vi "_interfacebrowser Build Interface Menu.vi"(5 "Tree":refnum<vi>, 7 "CtlRef":refnum<vi>, 9 "Coords":T1, 11 "Menu in":refnum<k9>) -> (3 "Discard?":bool)   [LabVIEW 2017, in "interfacebrowser.lvlib"]
uses:
  interfacebrowser.lvlib
  <vilib>/Utility/miscctls.llb/LVPoint32TypeDef.ctl
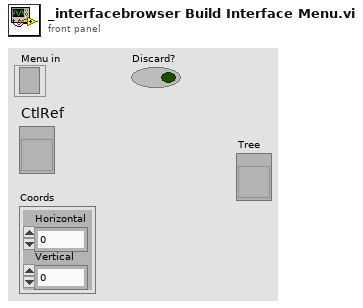
[diagram p1: front panel]
types:
  T1 = typedef "LVPoint32TypeDef.ctl" = cluster{"Horizontal":i32, "Vertical":i32}
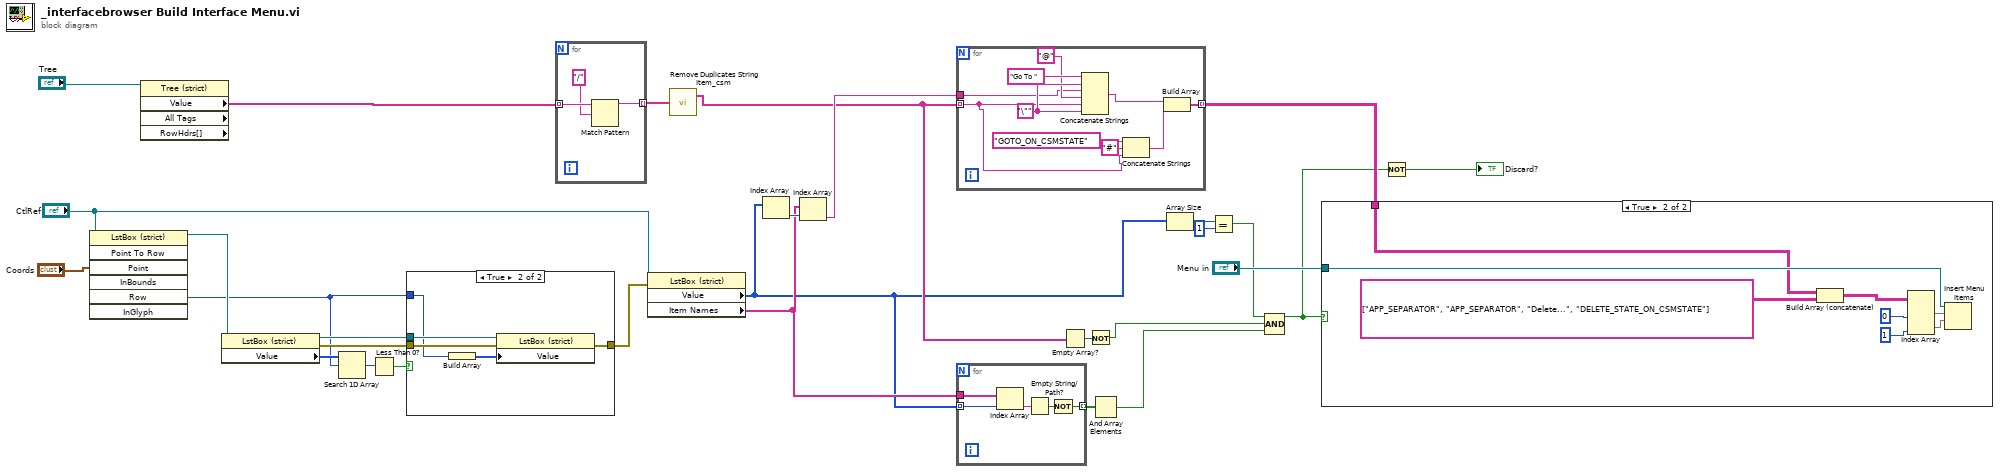
[diagram p0: block diagram]
diagram:
  n1 = invoke on="Invoke Node" class="LstBox (strict)" method="Point To Row"(reference="CtlRef", "Point"="Coords") -> (reference out=w26:refnum<vi>, "Row"=w19:i32)  [unwired: 5 in, 5 out]
  n2 = property on="Property Node" class="Tree (strict)" props=["Value", "All Tags", "RowHdrs[]"](reference="Tree") -> ("Value"=w14:string[])  [unwired: 1 in, 4 out]
  n3 = property on="Property Node" class="LstBox (strict)"(reference=w26) -> (reference out=w23:refnum<vi>, error out=w24:errorcluster, "Value"=w20:i32[])  [unwired: 1 in]
  n4 = Search 1D Array(1D array=w20, element=w19) -> (index of element=w25:i32)  [unwired: 1 in]
  n5 = Less Than 0?(x=w25) -> (x < 0?=w22:bool)
  n6 = case shown="True" w22 {
    tunnel: w24 -> [w30 w35]
    tunnel: w23 -> [_ w34]
    tunnel: w19 -> [_ w33]
    tunnel: [w30 w32] -> w21
    frame False {
    }
    frame True {
      n7 = Build Array(w33) -> (w31:i32[])
      n8 = property on="Property Node" class="LstBox (strict)"(reference=w34, error in=w35, "Value"=w31) -> (error out=w32:errorcluster)  [unwired: 1 out]
    }
  }
  n9 = for {
    tunnel: w14 -> [w38] mode=indexing
    tunnel: [w36] -> w13 mode=indexing
    n10 = Match Pattern(string=w38, regular expression="/") -> (before substring=w36:string)  [unwired: 1 in, 3 out]
  }
  n11 = property on="Property Node" class="LstBox (strict)"(reference="CtlRef", error in=w21) -> ("Value"=w9:i32[], "Item Names"=w10:string[])  [unwired: 2 out]
  n12 = call "Remove Duplicates String Item_csm.vi"("Input Array"=w13) -> ("Output Array"=w12:string[])  [unwired: 1 out]
  n13 = Index Array(array=w9) -> (element=w16:i32)  [unwired: 1 in]
  n14 = Index Array(array=w10, index=w16) -> (element=w15:string)
  n15 = for {
    tunnel: w12 -> [w39] mode=indexing
    tunnel: [w44] -> w17 mode=indexing
    tunnel: w15 -> [w42]
    w47 = "\"" ("string")
    n16 = Concatenate Strings("Go To " ("string"), w47, w42, "@" ("string"), w39, w47) -> (w46:string)
    n17 = Concatenate Strings("GOTO_ON_CSMSTATE", "#" ("string"), w39) -> (w41:string)
    n18 = Build Array(w46, w41) -> (w44:string[])
  }
  n19 = for {
    tunnel: w10 -> [w53]
    tunnel: w9 -> [w52] mode=indexing
    tunnel: [w49] -> w8 mode=indexing
    n20 = Index Array(array=w53, index=w52) -> (element=w51:string)
    n21 = Empty String/Path?(string/path=w51) -> (empty?=w50:bool)
    n22 = Not(x=w50) -> (.not. x?=w49:bool)
  }
  n23 = Empty Array?(array=w12) -> (empty?=w11:bool)
  n24 = Not(x=w11) -> (.not. x?=w7:bool)
  n25 = And Array Elements(Boolean array=w8) -> (logical AND=w6:bool)
  n26 = Array Size(array=w9) -> (size(s)=w5:i32)
  n27 = Equal?(x=w5, y=1) -> (x = y?=w3:bool)
  n28 = Compound Arithmetic op=AND(w3, w7, w6) -> (w2:bool)
  n29 = case shown="True" w2 {
    tunnel: "Menu in" -> [_ w61]
    tunnel: w17 -> [_ w54]
    frame False {
    }
    frame True {
      n30 = Build Array (concatenate)(w54, string[][] [["APP_SEPARATOR", "APP_SEPARATOR"], ["Delete...", "DELETE_STATE_ON_CSMSTATE"]] ("item names")) -> (w55:string[][])
      n31 = Index Array(array=w55, index (col) #1=0 ("disabled index (col)"), index (col) #2=1 ("index (col)")) -> (element #1=w59:string[], element #2=w58:string[])  [unwired: 2 in]
      n32 = Insert Menu Items(7:w58, 8:w59, 9:w61) -> ()  [unwired: 3 in, 3 out]
    }
  }
  n33 = Not(x=w2) -> (.not. x?=→"Discard?":bool)
